vi "巡线.vi"() -> ()   [LabVIEW 2018]
uses:
  <vilib>/vision/driver/IMAQdx.llb/IMAQdx Acquisition Mode.ctl
  <vilib>/vision/driver/IMAQdx.llb/IMAQdx Buffer Number Mode.ctl
  <vilib>/vision/Measure.llb/Edge Options.ctl
  <vilib>/vision/Measure.llb/Edge Polarity.ctl
  <vilib>/MakerHub/LINX/Public/Peripherals/Digital/Digital Write N Chans.vi
  <vilib>/MakerHub/LINX/Private/Local IO/LinxDigitalWrite.vi
  <vilib>/MakerHub/LINX/Public/Utilities/Check Channel.vi
  <vilib>/MakerHub/LINX/Public/Utilities/Open Serial.vi
  <vilib>/MakerHub/LINX/Private/Utilties/Generate Error.vi
  <vilib>/vision/NI_Vision_Development_Module.lvlib
  <vilib>/MakerHub/LINX/LMH-LINX.lvlib
  <vilib>/vision/driver/NI_Vision_Acquisition_Software.lvlib
panel:
  out "Error Out":errorcluster
  in  "Serial Port":refnum<visa-resource-name>="COM8"
  out "Image Out 3":T1(plugin-control)
  out "Location (Pixel).X":sgl
  out "InRange？":bool
  in  "Stop Button 2":bool
  in  "Session In 2":refnum<k21>="cam6" caption="IMAQdx Session"
  out "Image Out":T1(plugin-control)
  in  "DelayAdjust(ms)":dbl=0.04000000000000001 format="%#_13g"
  in  "lower limit":sgl=300.0
  in  "upper limit":sgl=500.0
  # "视 觉 寻 线 小 车"
  # "端口配置"
  # "实时显示"
  # "参数设置"
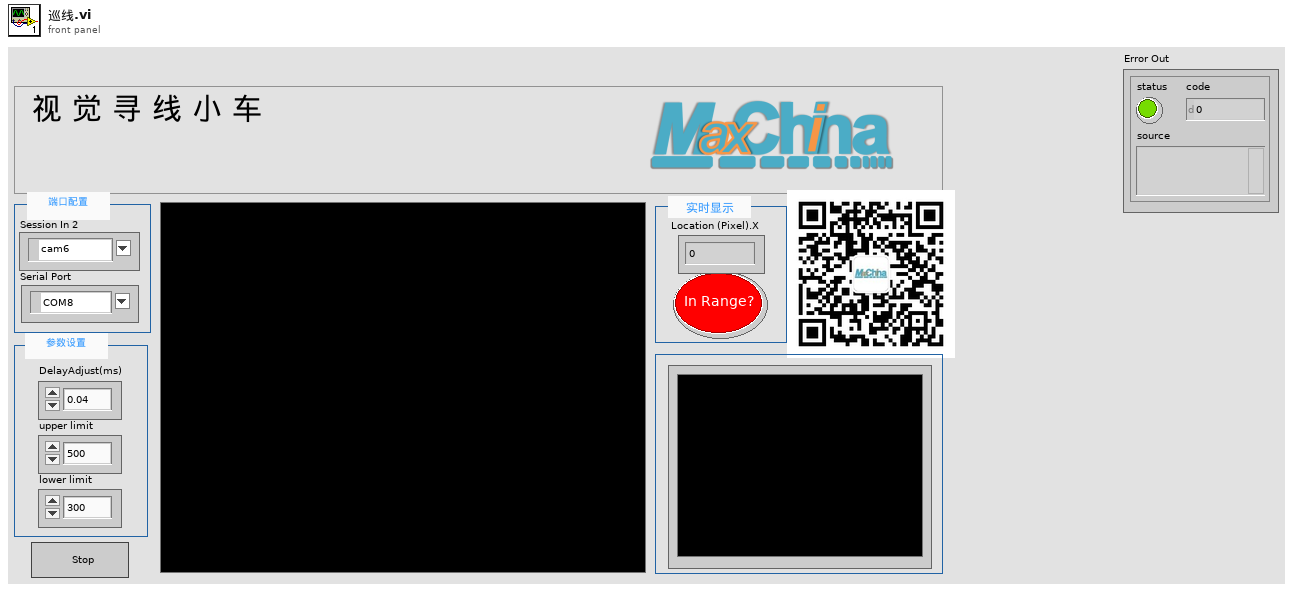
[diagram p1: front panel]
types:
  T1 = typedef "IMAQ Image.ctl" = refnum<image>
  T2 = typedef "NI_Vision_Acquisition_Software.lvlib/IMAQdx Acquisition Mode.ctl" = enum32{"One Shot", "Continuous"}
  T3 = typedef "Image Type" = u32
  T4 = cluster{"Global Rectangle":i32[], "Contours":cluster{"Contour Type":u32, "ROI Type":u32, "Points":i32[]}[]}
  T5 = typedef "IMAQdx.ctl" = refnum<k21>
  T6 = typedef "LMH-LINX.lvlib/LINX Ref.ctl" = cluster{"IO":T7, "Interface":T8, "LINX Device Config":T9}
  T7 = typedef "LMH-LINX.lvlib/Platform.ctl" = enum16{"Remote", "Local"}
  T8 = typedef "LMH-LINX.lvlib/Interface.ctl" = enum16{"Serial", "TCP"}
  T9 = typedef "LMH-LINX.lvlib/Device.lvlib/LINX Device Config.ctl" = cluster{"Interface":T8, "COM Port":refnum<visa-resource-name>, "TCP Configuration":T10, "Device Family":u8, "Device ID":u8, "Device Name":string, "TCP Ref":refnum<k5>, "Channels":T11}
  T10 = typedef "LMH-LINX.lvlib/Device.lvlib/TCP Config.ctl" = cluster{"IP Address":string, "Port":u16}
  T11 = typedef "LMH-LINX.lvlib/Channels.ctl" = cluster{"DI":u8[], "DO":u8[], "AI":u8[], "AO":u8[], "PWM":u8[], "QE":u8[], "UART":u8[], "I2C 2":u8[], "SPI":u8[], "CAN":u8[], "Servo":u8[], "AI Ref (V)":dbl, "AI Resolution (Bits)":u8, "AO Ref (V)":dbl, "AO Resolution (Bits)":u8}
  T12 = cluster{"Left":i32, "Top":i32, "Right":i32, "Bottom":i32}
  T13 = enum16{"Get First Edge", "Get First + Last Edge", "Get All Edges", "Get Best Edge"}
  T14 = typedef "Edge Options.ctl" = cluster{"Edge Polarity":T15, "Kernel Size":u32, "Width":u32, "Minimum Edge Strength":sgl, "Interpolation Type":enum32{"Zero Order", "Bilinear", "Quadratic", "Cubic", "Bilinear Fixed"}, "Data Processing Method":enum32{"Average", "Median"}}
  T15 = typedef "Edge Polarity.ctl" = u32
  T16 = typedef "NI_Vision_Acquisition_Software.lvlib/IMAQdx Buffer Number Mode.ctl" = enum32{"Next", "Last", "Buffer Number", "Every", "Last New"}
  T17 = typedef "Edge New.ctl" = cluster{"Location (Pixel)":cluster{"X":sgl, "Y":sgl}, "Location (Real-World)":cluster{"X":sgl, "Y":sgl}, "Distance (Pixel)":dbl, "Distance (Real-World)":dbl, "Strength":dbl, "Noise":dbl, "Rising?":bool}
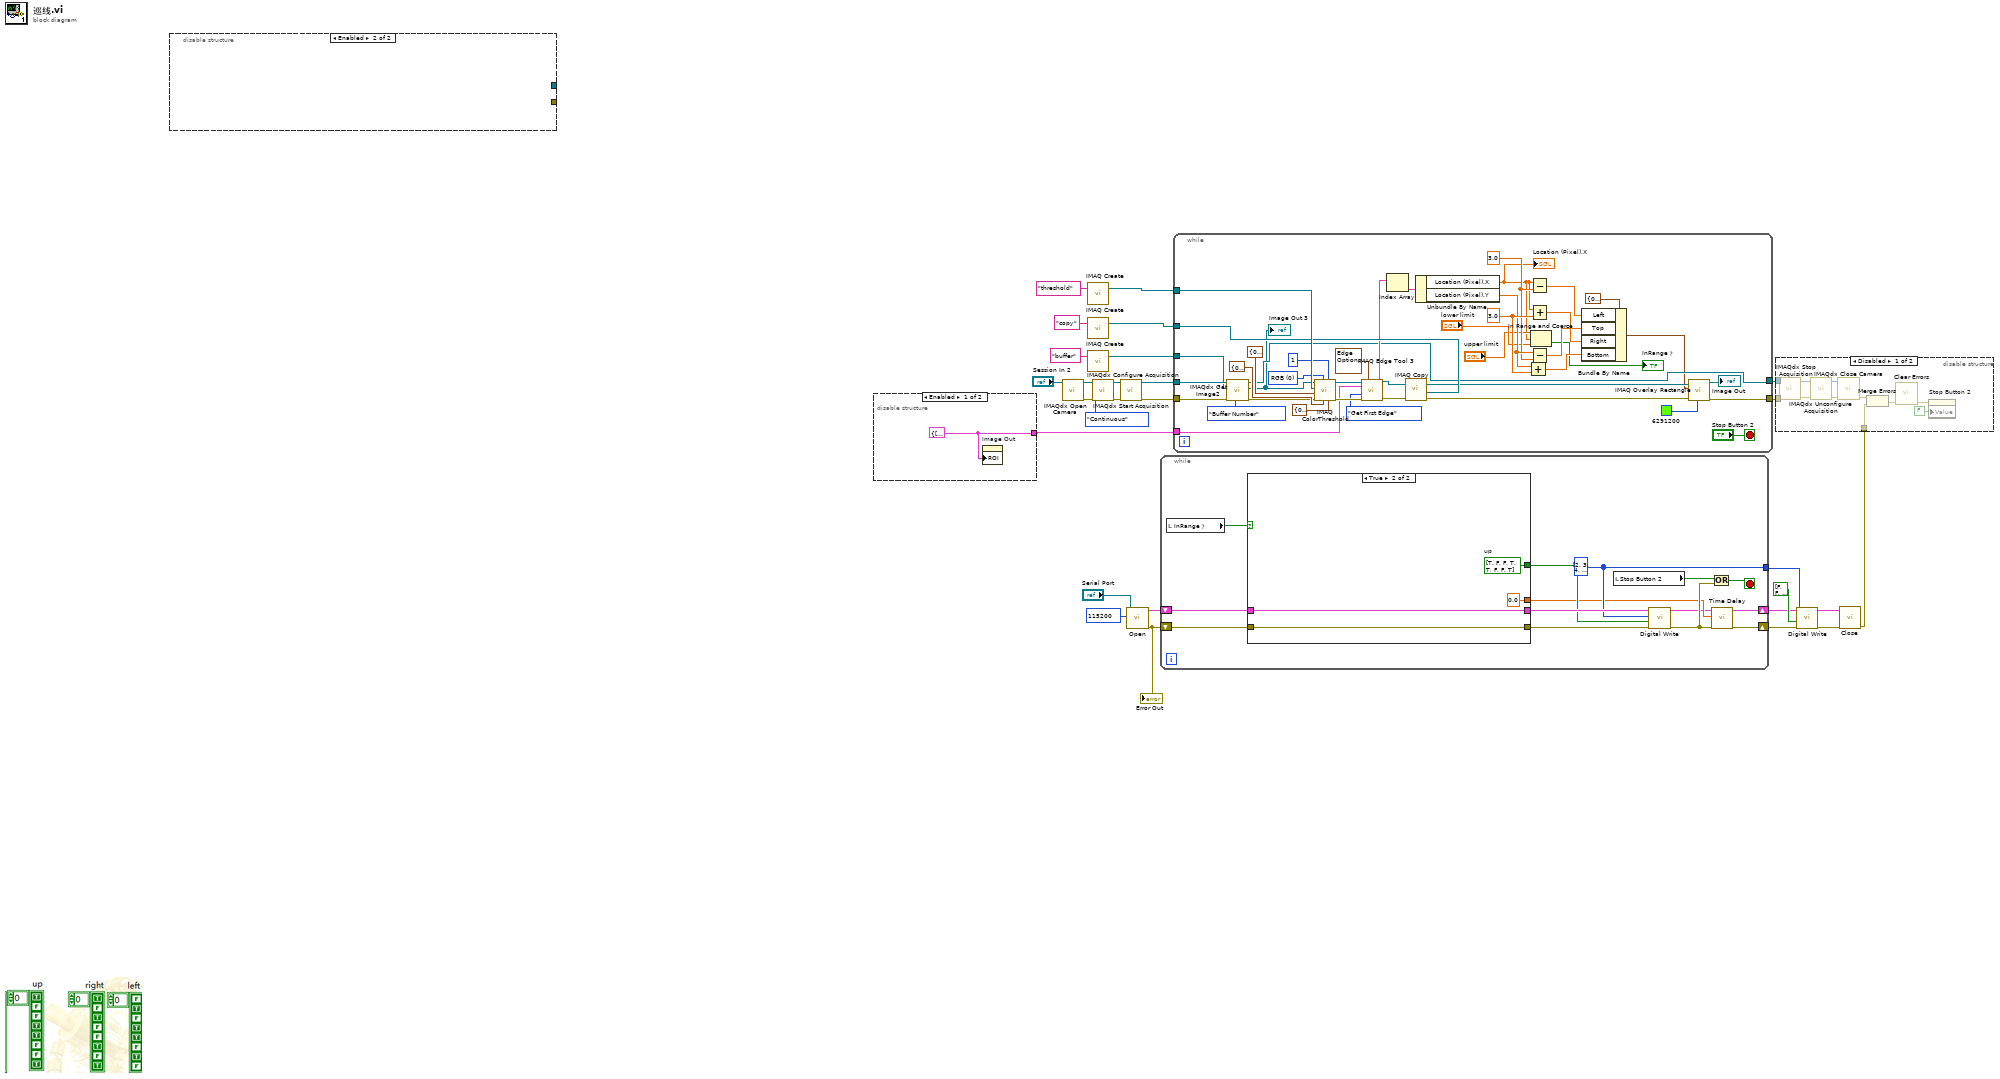
[diagram p0: block diagram]
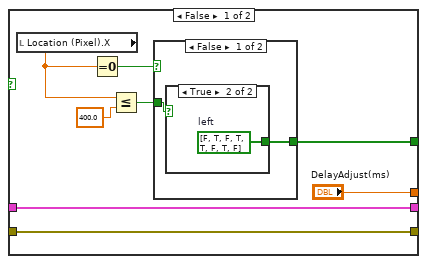
[diagram p3: hidden frame]
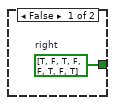
[diagram p4: hidden frame]
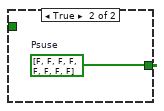
[diagram p5: hidden frame]
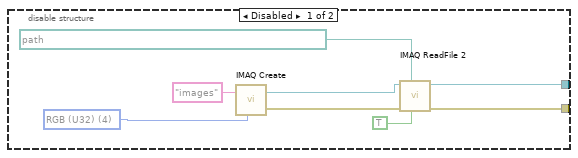
[diagram p6: hidden frame]
diagram:
  n1 = disable-structure shown="Enabled" {
    disable-tunnel: [w31 _] -> _
    disable-tunnel: [w30 _] -> _
    frame Disabled {
      w29 = T3 4 items=["Grayscale (U8)", "Grayscale (I16)", "Grayscale (SGL)", "Complex (CSG)", "RGB (U32)", "HSL (U32)", "RGB (U64)", "Grayscale (U16)"] ("Image Type")
      n2 = call "IMAQ Create"("Image Name"="images", "Image Type"=w29) -> ("New Image"=w32:T1, "error out"=w33:errorcluster)  [unwired: 3 in]
      n3 = call "IMAQ ReadFile 2"("Use File Path Image Type"=TRUE, "File Path"=path "D:/MaxChina/视觉项目/color/视觉巡线小车/right.jpg", "error in (no error)"=w33, "Image"=w32) -> ("error out"=w31:errorcluster, "Image Out"=w30:T1)  [unwired: 3 in, 3 out]
    }
    frame Enabled {
    }
  }
  n4 = disable-structure shown="Enabled" {
    disable-tunnel: [w37 _] -> w12
    frame Enabled {
      w37 = T4 {"Global Rectangle"=[2, 458, 640, 459], "Contours"=[{"Contour Type"=0, "ROI Type"=2, "Points"=[2, 458, 639, 458]}]} ("ROI")
      n5 = property on="Image Out" class="ImageControl"("ROI"=w37) -> ()  [unwired: 2 in, 2 out]
    }
    frame Disabled {
    }
  }
  n6 = call <vilib>:"IMAQdx Open Camera.vi"("Session In"="Session In 2") -> ("error out"=w21:errorcluster, "Session Out"=w24:T5)  [unwired: 9 in]
  n7 = call "IMAQ Create"("Image Name"="threshold") -> ("New Image"=w27:T1)  [unwired: 4 in, 1 out]
  n8 = call "IMAQ Create"("Image Name"="copy") -> ("New Image"=w25:T1)  [unwired: 4 in, 1 out]
  n9 = call "IMAQ Create"("Image Name"="buffer") -> ("New Image"=w18:T1)  [unwired: 4 in, 1 out]
  n10 = call <vilib>:"IMAQdx Configure Acquisition.vi"("error in"=w21, "Continuous?"=IMAQdx_Acquisition_Mode."Continuous", "Session In"=w24) -> ("error out"=w20:errorcluster, "Session Out"=w23:T5)  [unwired: 7 in]
  n11 = call <vilib>:"IMAQdx Start Acquisition.vi"("error in"=w20, "Session In"=w23) -> ("error out"=w19:errorcluster, "Session Out"=w22:T5)  [unwired: 8 in]
  n12 = call-poly <vilib>:"Open.vi"("Baud Rate Override"=u32 115200, "Serial Port"="Serial Port") -> ("Error Out"=w5:errorcluster, "LINX Resource"=w6:T6)  [unwired: 7 in, 1 out]
  "Error Out" <- w5
  n13 = while {
    shift-right: [w42] -> w8
    shift-left: w5 -> [w50]
    shift-right: [w40] -> w7
    shift-left: w6 -> [w48]
    tunnel: [w45] -> w4
    stop <- w49 stop-if-true
    w45 = u8[] [2, 3, 4, 5, 8, 9, 10, 11] ("DO Channels")
    n14 = local read "InRange？"() -> (w38:bool)
    n15 = case shown="True" w38 {
      tunnel: [w58 w67] -> w46
      tunnel: [w55 w66] -> w47
      tunnel: w50 -> [w58 w67]
      tunnel: w48 -> [w55 w66]
      tunnel: [w54 w65] -> w44
      tunnel: ["DelayAdjust(ms)" 0.0 ("Numeric Control")] -> w41
      frame False {
        n16 = local read "Location (Pixel).X"() -> (w53:sgl)
        n17 = Equal To 0?(x=w53) -> (x = 0?=w56:bool)
        n18 = Less Or Equal?(x=w53, y=sgl 400.0) -> (x <= y?=w57:bool)
        n19 = case shown="False" w56 {
          tunnel: [w60 w63] -> w54
          tunnel: w57 -> [w59 _]
          frame False {
            n20 = case shown="True" w59 {
              tunnel: [w61 w62] -> w60
              frame False {
                w61 = bool[] [TRUE, FALSE, TRUE, FALSE, FALSE, TRUE, FALSE, TRUE]  # right
              }
              frame True {
                w62 = bool[] [FALSE, TRUE, FALSE, TRUE, TRUE, FALSE, TRUE, FALSE]  # left
              }
            }
          }
          frame True {
            w63 = bool[] [FALSE, FALSE, FALSE, FALSE, FALSE, FALSE, FALSE, FALSE]  # Psuse
          }
        }
      }
      frame True {
        w65 = bool[] [TRUE, FALSE, FALSE, TRUE, TRUE, FALSE, FALSE, TRUE]  # up
      }
    }
    n21 = local read "Stop Button 2"() -> (w39:bool)
    n22 = call-poly <vilib>:"Digital Write.vi"("Error In"=w46, "Values"=w44, "DO Channels"=w45, "LINX Resource"=w47) -> ("Error Out"=w43:errorcluster, "LINX Resource"=w40:T6)  [unwired: 6 in]
    n23 = Or(x=w39, y=w43) -> (x .or. y?=w49:bool)
    n24 = call "Time Delay"("error in (no error)"=w43, "Delay Time (s)"=w41) -> ("error out"=w42:errorcluster)  [unwired: 9 in]
  }
  n25 = while {
    tunnel: w27 -> [w109]
    tunnel: w25 -> [w99]
    tunnel: w22 -> [w85]
    tunnel: w19 -> [w84]
    tunnel: w18 -> [w83]
    tunnel: [w82] -> w15
    tunnel: [w69] -> w14
    tunnel: w12 -> [w75]
    stop <- "Stop Button 2" stop-if-true
    w90 = sgl 3.0 ("y")
    w93 = sgl 3.0 ("y")
    w107 = u16 0 items=["RGB", "HSL", "HSV", "HSI"] ("Color Mode")
    n26 = call <vilib>:"IMAQdx Get Image2.vi"("Buffer Number Mode (Next)"=IMAQdx_Buffer_Number_Mode."Buffer Number", "error in"=w84, "Image In"=w83, "Session In"=w85) -> ("error out"=w81:errorcluster, "Image Out"=w79:T1, "Session Out"=w82:T5)  [unwired: 4 in, 1 out]
    "Image Out 3" <- w79
    n27 = call "IMAQ ColorThreshold"("Blue or Luma or Val or Inten Range"=cluster{"Lower value":i32, "Upper value":i32} {"Lower value"=0, "Upper value"=21}, "Replace Value"=1, "Green or Sat Range"=cluster{"Lower value":i32, "Upper value":i32} {"Lower value"=0, "Upper value"=57}, "Color Mode"=w107, "error in (no error)"=w81, "Red or Hue Range"=cluster{"Lower value":i32, "Upper value":i32} {"Lower value"=0, "Upper value"=10}, "Image Dst"=w109, "Image Src"=w79) -> ("error out"=w103:errorcluster, "Image Dst Out"=w102:T1)  [unwired: 2 in]
    n28 = call "IMAQ Edge Tool 3"("Image"=w102, "Edge Options"=T14 {"Edge Polarity"=0, "Kernel Size"=3, "Width"=1, "Minimum Edge Strength"=1.0, "Interpolation Type"=enum."Bilinear Fixed", "Data Processing Method"=enum."Median"}, "ROI Descriptor"=w75, "Process"=T13."Get First Edge", "error in (no error)"=w103) -> ("Image (duplicate)"=w100:T1, "Edge Information"=w86:T17[], "error out"=w71:errorcluster)  [unwired: 6 in, 2 out]
    n29 = Index Array(array=w86) -> (element=w97:T17)  [unwired: 1 in]
    n30 = call "IMAQ Copy"("error in (no error)"=w71, "Image Dst"=w99, "Image Src"=w100) -> ("error out"=w70:errorcluster, "Image Dst Out"=w98:T1)  [unwired: 3 in]
    n31 = Unbundle By Name(w97) -> ("Location (Pixel).X"=w72:sgl, "Location (Pixel).Y"=w91:sgl)
    "Location (Pixel).X" <- w72
    n32 = Add(x=w91, y=w93) -> (x+y=w94:sgl)
    n33 = Subtract(x=w72, y=w90) -> (x-y=w92:sgl)
    n34 = Add(x=w72, y=w93) -> (x+y=w95:sgl)
    n35 = Subtract(x=w91, y=w90) -> (x-y=w89:sgl)
    n36 = In Range and Coerce(upper limit="upper limit", x=w72, lower limit="lower limit") -> (In Range?=→"InRange？":bool)  [unwired: 1 out]
    n37 = Bundle By Name(cluster=T12 {"Left"=0, "Top"=0, "Right"=10, "Bottom"=10} ("Rectangle"), "Left"=w92, "Top"=w89, "Right"=w95, "Bottom"=w94) -> (w68:T12)
    n38 = call "IMAQ Overlay Rectangle"("Color"=u32 6291200, "error in (no error)"=w70, "Rectangle"=w68, "Image"=w98) -> ("error out"=w69:errorcluster, "Image Out"=→"Image Out":T1)  [unwired: 6 in]
  }
  n39 = call-poly <vilib>:"Digital Write.vi"("Error In"=w8, "Values"=bool[] [FALSE, FALSE, FALSE, FALSE, FALSE, FALSE, FALSE, FALSE], "DO Channels"=w4, "LINX Resource"=w7) -> ("Error Out"=w9:errorcluster, "LINX Resource"=w10:T6)  [unwired: 6 in]
  n40 = call <vilib>:"Close.vi"("Error In"=w9, "LINX Resource"=w10) -> ("Error Out"=w13:errorcluster)  [unwired: 9 in]
  n41 = disable-structure shown="Disabled" {
    disable-tunnel: w15 -> [w120 _]
    disable-tunnel: w14 -> [w119 _]
    disable-tunnel: w13 -> [w113 _]
    frame Disabled {
      n42 = call <vilib>:"IMAQdx Stop Acquisition.vi"("error in"=w119, "Session In"=w120) -> ("error out"=w118:errorcluster, "Session Out"=w115:T5)  [unwired: 8 in]
      n43 = call <vilib>:"IMAQdx Unconfigure Acquisition.vi"("error in"=w118, "Session In"=w115) -> ("error out"=w117:errorcluster, "Session Out"=w116:T5)  [unwired: 8 in]
      n44 = call <vilib>:"IMAQdx Close Camera.vi"("error in"=w117, "Session In"=w116) -> ("error out"=w114:errorcluster)  [unwired: 9 in]
      n45 = Merge Errors(w114, w113) -> (w112:errorcluster)
      n46 = call <vilib>:"Clear Errors.vi"("error in (no error)"=w112) -> ("error out"=w110:errorcluster)  [unwired: 5 in, 1 out]
      n47 = property on="Stop Button 2" class="Bool (strict)"(error in=w110, "Value"=FALSE ("stop")) -> ()  [unwired: 1 in, 2 out]
    }
    frame Enabled {
    }
  }
